vi "XML - Get relative Configuration LLB path.vi"(8 "error in (no error)":errorcluster, 11 "CD Wizard - Internal Data":T1) -> (0 "error out":errorcluster, 3 "Relative Configuration LLB path":path)   [LabVIEW 2015]
doc: "Create the relative path for the Configuration LLB based on the name and execution mode of the new custom device."
uses:
  TypDef/CD Wizard - Internal data.ctl
  TypDef/CD Wizard - Execution Mode.ctl
  TypDef/CD Wizard - Extra Page Name and GUID.ctl
  Constants/Constants TypDef/Build Spec System Explorer.ctl
  Constants/Build Spec System Explorer.vi
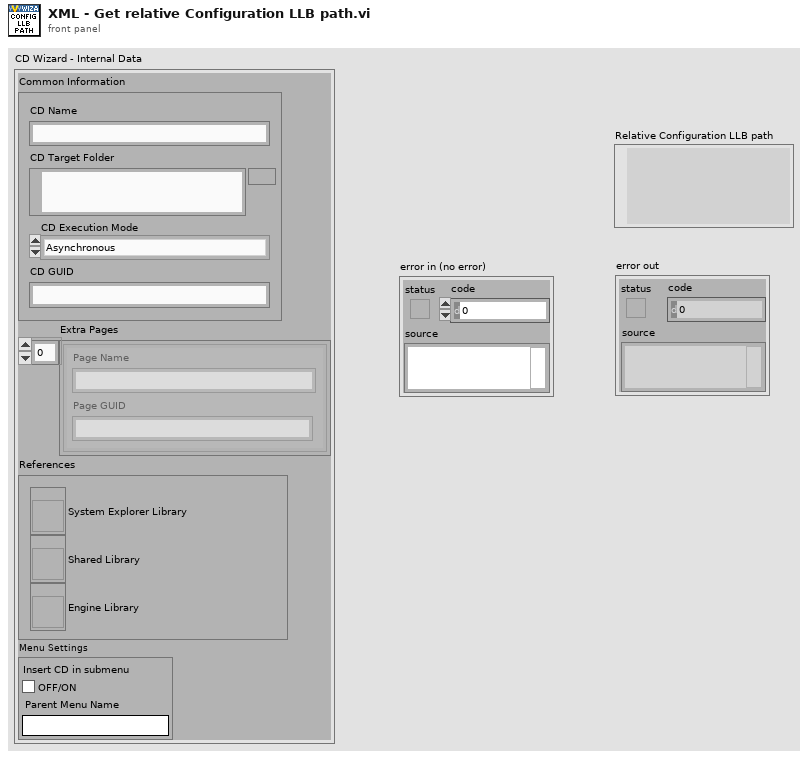
[diagram p1: front panel]
types:
  T1 = typedef "CD Wizard - Internal data.ctl" = cluster{"Common Information":cluster{"CD Name":string, "CD Target Folder":path, "CD Execution Mode":T2, "CD GUID":string}, "Extra Pages":T3[], "References":cluster{"System Explorer Library":refnum<vi>, "Shared Library":refnum<vi>, "Engine Library":refnum<vi>}, "Menu Settings":cluster{"Insert CD in submenu":bool, "Parent Menu Name":string}}
  T2 = typedef "CD Wizard - Execution Mode.ctl" = enum16{"Asynchronous", "Inline HW Interface", "Inline Model Interface", "Inline Timing and Sync", "Asynchronous Timing and Sync"}
  T3 = typedef "CD Wizard - Extra Page Name and GUID.ctl" = cluster{"Page Name":string, "Page GUID":string}
  T4 = typedef "Build Spec System Explorer.ctl" = enum16{"Destinations.LLBFileName"}
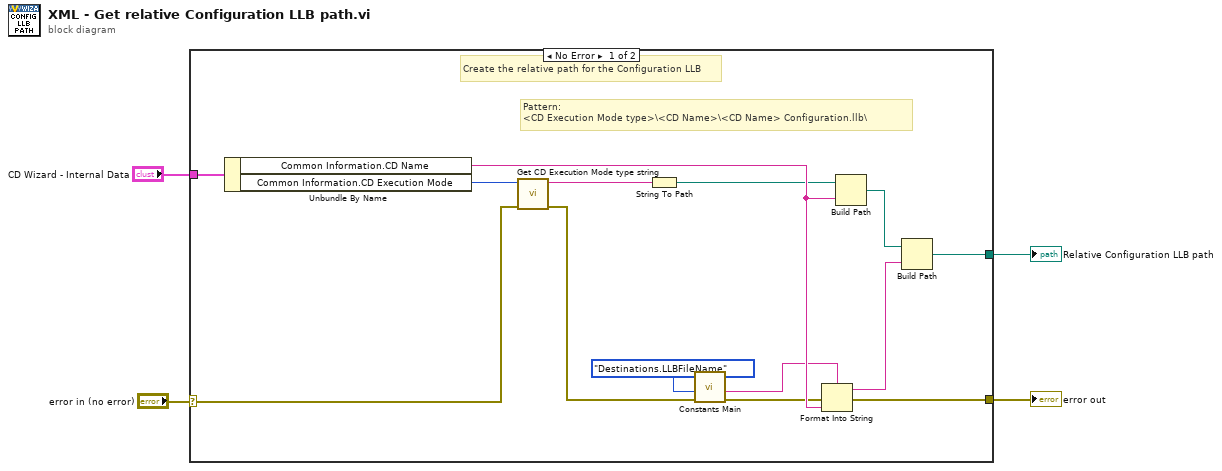
[diagram p0: block diagram]
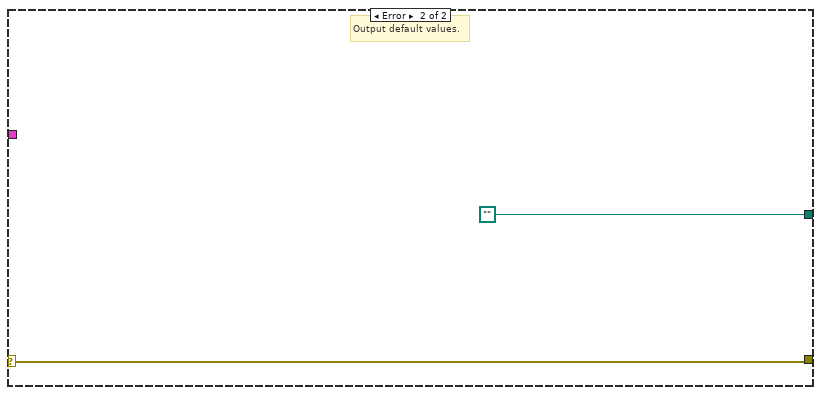
[diagram p2: hidden frame]
diagram:
  n1 = case shown="No Error" "error in (no error)" {
    selector: "error in (no error)" -> [w5 w20]
    tunnel: [w10 w20] -> w3
    tunnel: [w9 path ""] -> w1
    tunnel: "CD Wizard - Internal Data" -> [w11 _]
    frame No Error {
      # "Pattern:\n<CD Execution Mode type>\\<CD Name>\\<CD Name> Configuration.llb\\"
      # "Create the relative path for the Configuration LLB"
      n2 = Unbundle By Name(w11) -> ("Common Information.CD Name"=w18:string, "Common Information.CD Execution Mode"=w7:T2)
      n3 = call "Get CD Execution Mode type string.vi"("error in (no error)"=w5, "CD Execution Mode"=w7) -> ("error out"=w6:errorcluster, "Execution Mode type"=w8:string)  [unwired: 8 in]
      n4 = String To Path(string=w8) -> (path=w12:path)
      n5 = call-poly "Constants Main.vi"("error in (no error)"=w6, "Action"=Build_Spec_System_Explorer."Destinations.LLBFileName") -> ("error out"=w15:errorcluster, "Output"=w16:string)  [unwired: 8 in]
      n6 = Format Into String(format string=w16, error in=w15, w18) -> (resulting string=w17:string, error out=w10:errorcluster)  [unwired: 1 in]
      n7 = Build Path(base path=w12, name or relative path=w18) -> (appended path=w13:path)
      n8 = Build Path(base path=w13, name or relative path=w17) -> (appended path=w9:path)
    }
    frame Error {
      # "Output default values."
    }
  }
  "error out" <- w3
  "Relative Configuration LLB path" <- w1
